vi "DefenderNormal.vi"(4 "Enemy Robots":T1, 5 "total":i32, 6 "balls":T4[](array[typedef]), 7 "cont old":dbl, 8 "ball old":dbl[](array[numeric]), 9 "Field Size in":T5, 10 "Numeric":i32, 11 "Our Robot in":T1) -> (1 "cont new":dbl, 2 "new ball":dbl[](array[numeric]), 3 "Robot out":T1)   [LabVIEW 2016]
uses:
  Core/AI Robot.ctl
  Functions Enum.ctl
  Core/Field Size.ctl
  Core/AI Ball.ctl
  <vilib>/Analysis/Matrix/Datatypes/RealMatrix.ctl
  <vilib>/Analysis/NI_AALBase.lvlib
  <vilib>/Analysis/baseanly.llb/Real A x B.vi
  <vilib>/Analysis/Matrix/NI_Matrix.lvlib
panel:
  in  "min dist to kick":dbl=195.0 format="%#_13g"
  in  "D max":dbl=400.0
  in  "D min":dbl=400.0
  in  "array":dbl[](array[numeric])
  out "fora?":bool
  in  "matrix":T3
  in  "y":dbl
  in  "raio robo":dbl=-90.0 format="%#_13g"
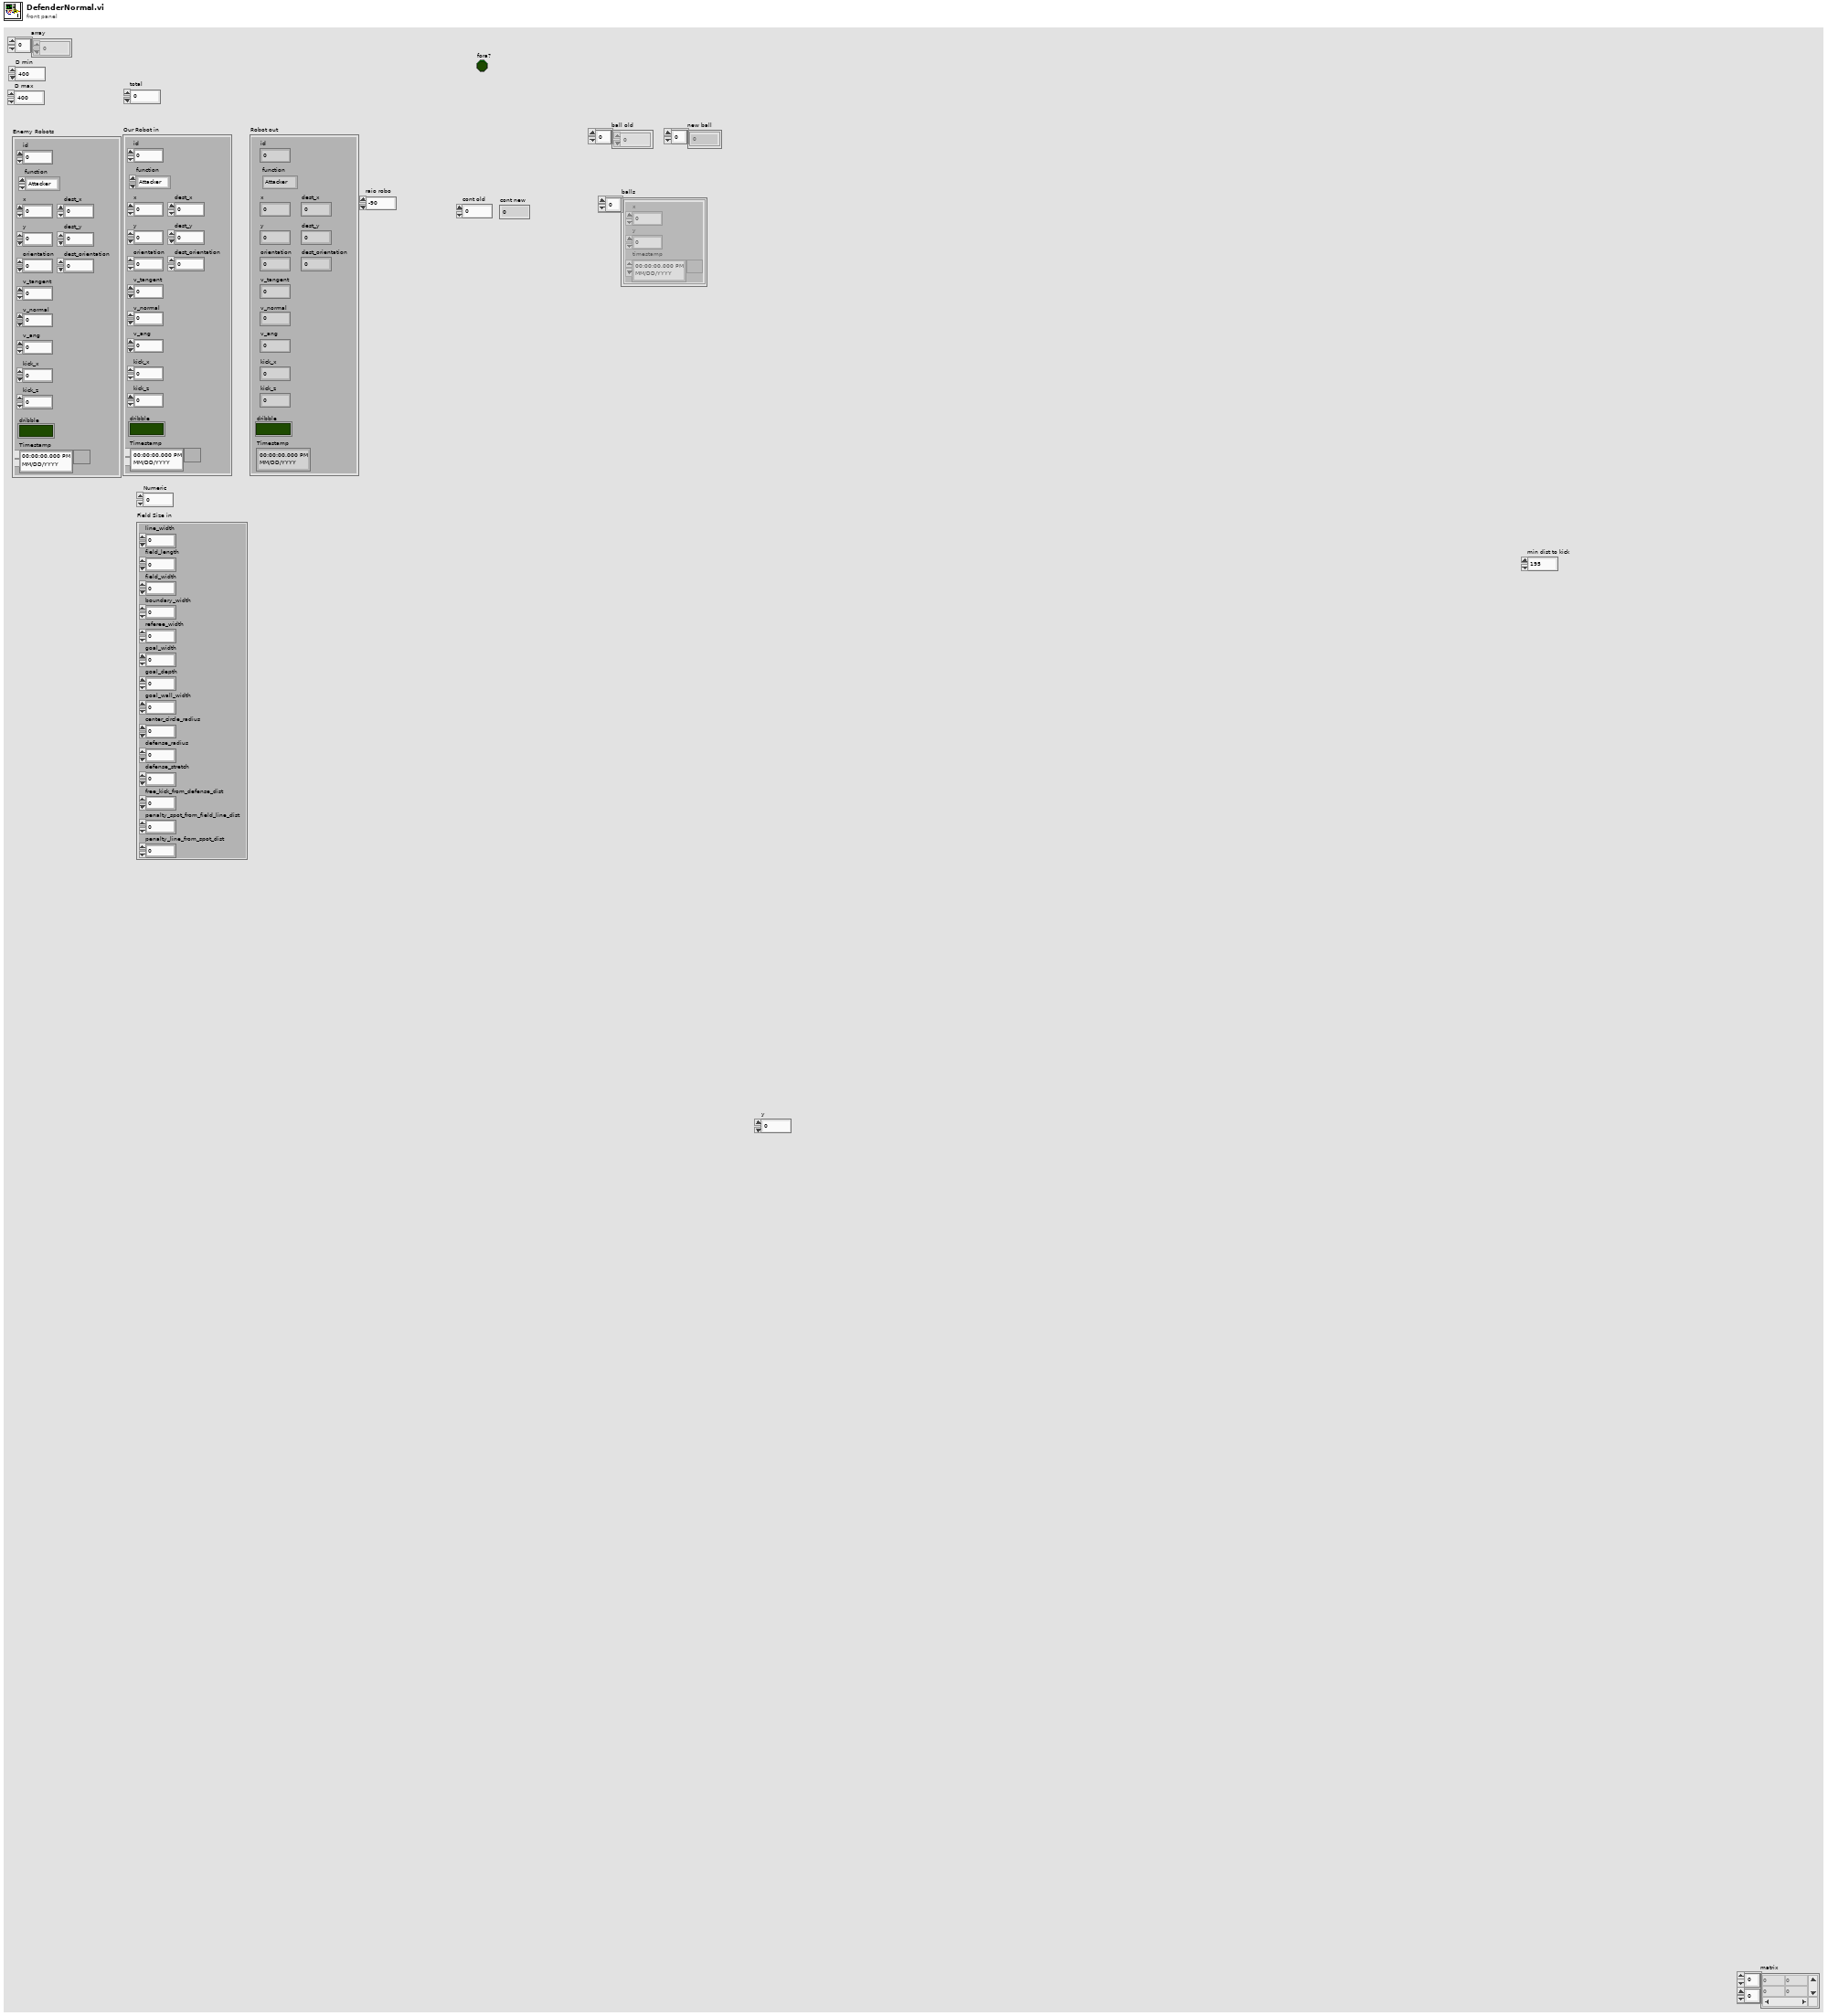
[diagram p1: front panel]
types:
  T1 = typedef "AI Robot.ctl" = cluster{"id":u32, "function":T2, "x":dbl, "y":dbl, "orientation":dbl, "v_tangent":dbl, "v_normal":dbl, "v_ang":dbl, "kick_x":dbl, "kick_z":dbl, "dribble":bool, "Timestamp":timestamp, "dest_x":dbl, "dest_y":dbl, "dest_orientation":dbl}
  T2 = typedef "Functions Enum.ctl" = enum16{"Attacker", "Goalie", "Defender", "Striker", "Goto 0", "Dummy", "ZigZag"}
  T3 = typedef "NI_Matrix.lvlib/RealMatrix.ctl" = dbl[][]
  T4 = typedef "AI Ball.ctl" = cluster{"x":dbl, "y":dbl, "timestamp":timestamp}
  T5 = typedef "Field Size.ctl" = cluster{"line_width":u32, "field_length":u32, "field_width":u32, "boundary_width":u32, "referee_width":u32, "goal_width":u32, "goal_depth":u32, "goal_wall_width":u32, "center_circle_radius":u32, "defense_radius":u32, "defense_stretch":u32, "free_kick_from_defense_dist":u32, "penalty_spot_from_field_line_dist":u32, "penalty_line_from_spot_dist":u32}
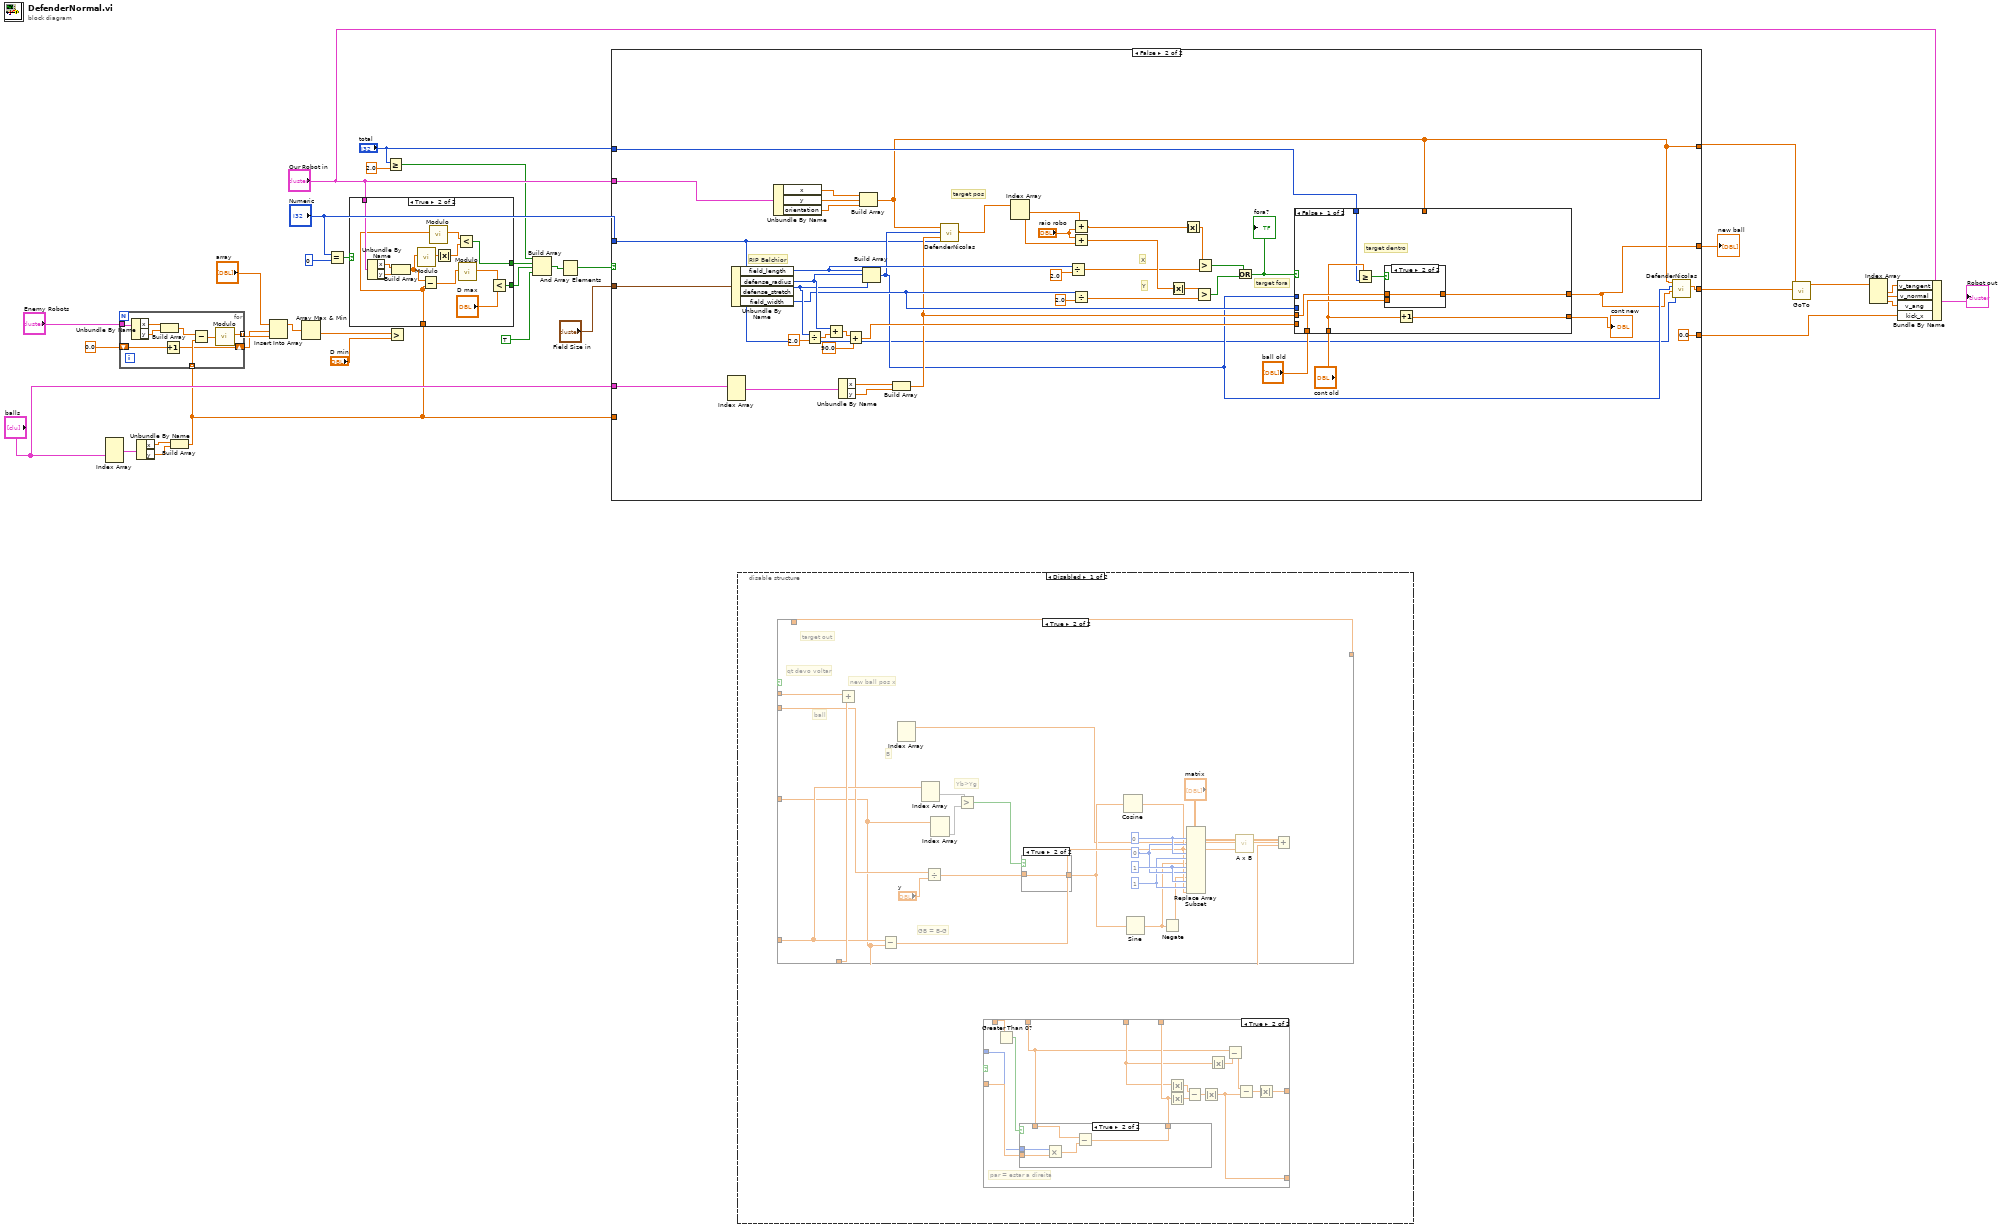
[diagram p0: block diagram]
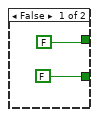
[diagram p2: hidden frame]
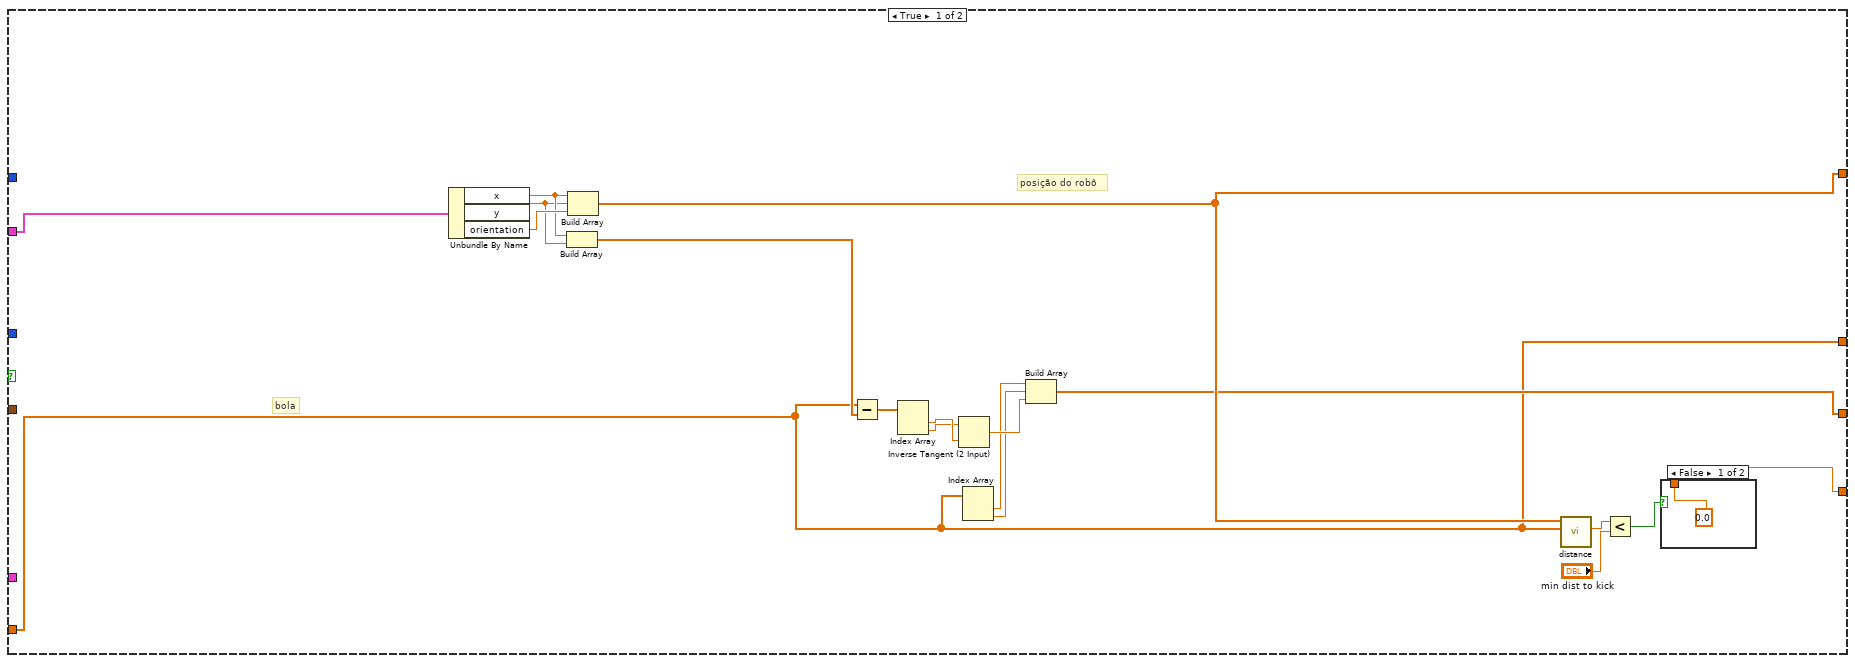
[diagram p3: hidden frame]
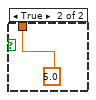
[diagram p4: hidden frame]
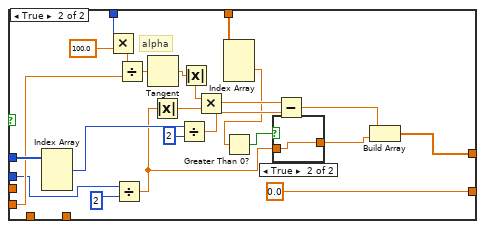
[diagram p6: hidden frame]
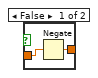
[diagram p7: hidden frame]
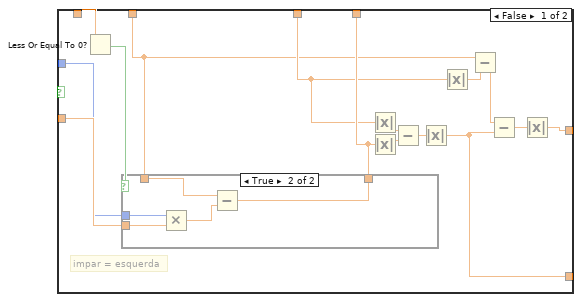
[diagram p8: hidden frame]
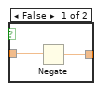
[diagram p12: hidden frame]
diagram:
  n1 = Index Array(array="balls") -> (element #1=w28:T4)  [unwired: 3 in, 2 out]
  n2 = Unbundle By Name(w28) -> ("x"=w5:dbl, "y"=w27:dbl)
  n3 = Build Array(w5, w27) -> (w6:dbl[])
  n4 = for {
    tunnel: "Enemy Robots" -> [w44]
    tunnel: w6 -> [w39] mode=indexing
    tunnel: [w38] -> w12 mode=indexing
    shift-right: [w36] -> w10
    shift-left: 0.0 -> [w37]
    n5 = Unbundle By Name(w44) -> ("x"=w43:dbl, "y"=w42:dbl)
    n6 = Build Array(w43, w42) -> (w41:dbl[])
    n7 = Increment(x=w37) -> (x+1=w36:dbl)
    n8 = Subtract(x=w41, y=w39) -> (x-y=w40:dbl[])
    n9 = call "Modulo.vi"("2D vector"=w40) -> ("Modulo"=w38:dbl)  [unwired: 10 in]
  }
  n10 = Insert Into Array(array="array", index=w10, new element=w12) -> (w9:dbl[])
  n11 = Array Max & Min(array=w9) -> (min value=w8:dbl)  [unwired: 3 out]
  n12 = Equal?(x="Numeric", y=0) -> (x = y?=w22:bool)
  n13 = case shown="True" w22 {
    tunnel: "Our Robot in" -> [_ w59]
    tunnel: [FALSE w55] -> w19
    tunnel: w6 -> [_ w49]
    tunnel: [FALSE w51] -> w3
    frame False {
    }
    frame True {
      n14 = Unbundle By Name(w59) -> ("x"=w53:dbl, "y"=w58:dbl)
      n15 = Build Array(w53, w58) -> (w47:dbl[])
      n16 = call "Modulo.vi"("2D vector"=w47) -> ("Modulo"=w48:dbl)  [unwired: 10 in]
      n17 = Subtract(x=w47, y=w49) -> (x-y=w54:dbl[])
      n18 = call "Modulo.vi"("2D vector"=w49) -> ("Modulo"=w50:dbl)  [unwired: 10 in]
      n19 = Absolute Value(x=w48) -> (abs(x)=w52:dbl)
      n20 = Less?(x=w50, y=w52) -> (x < y?=w51:bool)
      n21 = call "Modulo.vi"("2D vector"=w54) -> ("Modulo"=w57:dbl)  [unwired: 10 in]
      n22 = Less?(x=w57, y="D max") -> (x < y?=w55:bool)
    }
  }
  n23 = Greater Or Equal?(x="total", y=2.0) -> (x >= y?=w4:bool)
  n24 = Greater?(x=w8, y="D min") -> ()  [unwired: 1 out]
  n25 = Build Array(w4, w3, w19, TRUE ("element")) -> (w18:bool[])
  n26 = And Array Elements(Boolean array=w18) -> (logical AND=w17:bool)
  n27 = case shown="False" w17 {
    tunnel: "Our Robot in" -> [w61 w112]
    tunnel: "Field Size in" -> [_ w110]
    tunnel: "balls" -> [_ w102]
    tunnel: [w64 w80] -> w30
    tunnel: "Numeric" -> [_ w81]
    tunnel: [w73 w84] -> w29
    tunnel: "total" -> [_ w89]
    tunnel: [w74 0.0] -> w16
    tunnel: w6 -> [w60 _]
    tunnel: [w60 w82] -> w2
    frame True {
      # "posição do robô"
      # "bola"
      n28 = Unbundle By Name(w61) -> ("x"=w71:dbl, "y"=w70:dbl, "orientation"=w72:dbl)
      n29 = Build Array(w71, w70) -> (w69:dbl[])
      n30 = Build Array(w71, w70, w72) -> (w73:dbl[])
      n31 = Subtract(x=w60, y=w69) -> (x-y=w68:dbl[])
      n32 = Index Array(array=w68) -> (element #1=w66:dbl, element #2=w65:dbl)  [unwired: 2 in]
      n33 = Inverse Tangent (2 Input)(1:w66, 2:w65) -> (0:w67:dbl)
      n34 = Index Array(array=w60) -> (element #1=w63:dbl, element #2=w62:dbl)  [unwired: 2 in]
      n35 = Build Array(w63, w62, w67) -> (w64:dbl[])
      n36 = call "distance.vi"("target pos"=w60, "obj pos"=w73) -> ("sqrt(x)"=w77:dbl)  [unwired: 9 in]
      n37 = Less?(x=w77, y="min dist to kick") -> (x < y?=w76:bool)
      n38 = case shown="False" w76 {
        tunnel: [0.0 5.0] -> w74
        frame False {
        }
        frame True {
        }
      }
    }
    frame False {
      # "RIP Belchior"
      # "target fora"
      # "Y"
      # "X"
      # "target pos"
      n39 = Index Array(array=w102) -> (element #1=w123:T4)  [unwired: 3 in, 2 out]
      n40 = Unbundle By Name(w110) -> ("field_length"=w107:u32, "defense_radius"=w97:u32, "defense_stretch"=w94:u32, "field_width"=w90:u32)
      n41 = Unbundle By Name(w112) -> ("x"=w108:dbl, "y"=w104:dbl, "orientation"=w103:dbl)
      n42 = Divide(x=w94, y=2.0) -> (x/y=w95:dbl)
      n43 = Add(x=w97, y=w95) -> (x+y=w92:dbl)
      n44 = Unbundle By Name(w123) -> ("x"=w113:dbl, "y"=w109:dbl)
      n45 = Add(x=w92, y=90.0) -> (x+y=w93:dbl)
      n46 = Build Array(w108, w104, w103) -> (w84:dbl[])
      n47 = Build Array(w107, w97, w94) -> (w83:u32[])
      n48 = Build Array(w113, w109) -> (w86:dbl[])
      n49 = call "DefenderNicolas.vi"("R"=w84, "Field"=w83, "Ball"=w86, "Numeric"=w81) -> ("target"=w85:dbl[])  [unwired: 6 in]
      n50 = Index Array(array=w85) -> (element #1=w106:dbl, element #2=w105:dbl)  [unwired: 2 in]
      n51 = Divide(x=w107, y=2.0) -> (x/y=w101:dbl)
      n52 = Add(x=w106, y="raio robo") -> (x+y=w111:dbl)
      n53 = Add(x="raio robo", y=w105) -> (x+y=w114:dbl)
      n54 = Divide(x=w90, y=2.0) -> (x/y=w116:dbl)
      n55 = Absolute Value(x=w114) -> (abs(x)=w119:dbl)
      n56 = Absolute Value(x=w111) -> (abs(x)=w120:dbl)
      n57 = Greater?(x=w119, y=w116) -> (0:w117:bool)
      n58 = Greater?(x=w120, y=w101) -> (0:w118:bool)
      n59 = Or(x=w118, y=w117) -> (x .or. y?=w100:bool)
      "fora?" <- w100
      n60 = case shown="False" w100 {
        tunnel: w86 -> [w128 _]
        tunnel: [w129 w152] -> w82
        tunnel: "ball old" -> [w127 _]
        tunnel: "cont old" -> [w125 _]
        tunnel: [w130 0.0] -> w98
        tunnel: w83 -> [_ w154]
        tunnel: w93 -> [_ w148]
        tunnel: w89 -> [w124 w151]
        tunnel: w90 -> [_ w141]
        tunnel: w84 -> [_ w137]
        frame False {
          # "target dentro"
          n61 = Greater Or Equal?(x=w125, y=w124) -> (x >= y?=w126:bool)
          n62 = case shown="True" w126 {
            tunnel: [w131 w132] -> w129
            tunnel: w128 -> [_ w132]
            tunnel: w127 -> [w131 _]
            frame False {
            }
            frame True {
            }
          }
          n63 = Increment(x=w125) -> (x+1=w130:dbl)
        }
        frame True {
          # "alpha"
          n64 = Index Array(array=w154) -> (element #1=w139:u32)  [unwired: 3 in, 2 out]
          n65 = Multiply(x=w151, y=100.0) -> (x*y=w149:dbl)
          n66 = Divide(x=w141, y=u32 2) -> (x/y=w134:dbl)
          n67 = Divide(x=w149, y=w148) -> (x/y=w146:dbl)
          n68 = Tangent(1:w146) -> (0:w145:dbl)
          n69 = Absolute Value(x=w134) -> (abs(x)=w144:dbl)
          n70 = Divide(x=w139, y=u32 2) -> (x/y=w140:dbl)
          n71 = Absolute Value(x=w145) -> (abs(x)=w147:dbl)
          n72 = Multiply(x=w147, y=w144) -> (x*y=w143:dbl)
          n73 = Index Array(array=w137) -> (element #2=w136:dbl)  [unwired: 3 in, 2 out]
          n74 = Greater Than 0?(x=w136) -> (x > 0?=w135:bool)
          n75 = case shown="True" w135 {
            tunnel: w134 -> [w157 w158]
            tunnel: [w156 w158] -> w133
            frame False {
              n76 = Negate(x=w157) -> (-x=w156:dbl)
            }
            frame True {
            }
          }
          n77 = Subtract(x=w143, y=w140) -> (x-y=w142:dbl)
          n78 = Build Array(w142, w133) -> (w152:dbl[])
        }
      }
      "cont new" <- w98
      n79 = call "DefenderNicolas.vi"("R"=w84, "Field"=w83, "Ball"=w82, "Numeric"=w81) -> ("target"=w80:dbl[])  [unwired: 6 in]
    }
  }
  "new ball" <- w2
  n80 = disable-structure shown="Disabled" {
    frame Disabled {
      n81 = case shown="True" {
        selector: _ -> [_ _]
        tunnel: _ -> [_ w225]
        tunnel: _ -> [_ w224]
        tunnel: _ -> [_ w206]
        tunnel: _ -> [_ w207]
        tunnel: _ -> [_ w204]
        tunnel: [w201 w202] -> _
        tunnel: _ -> [w201 w202]
        frame False {
        }
        frame True {
          w220 = 1
          w221 = 0
          w222 = 1
          w223 = 0
          # "B"
          # "Yb>Yg"
          # "GB = B-G"
          # "new ball pos x"
          # "qt devo voltar"
          # "ball"
          # "target out"
          n82 = Add(x=w224, y=w225) -> ()  [unwired: 1 out]
          n83 = Subtract(x=w207, y=w204) -> (x-y=w215:dbl)
          n84 = Index Array(array=w207) -> (element #2=w214)  [unwired: 2 in, 1 out]
          n85 = Divide(x=w206, y="y") -> (x/y=w211:dbl)
          n86 = Index Array(array=w204) -> (element #2=w213)  [unwired: 2 in, 1 out]
          n87 = Greater?(x=w214, y=w213) -> (0:w212:bool)
          n88 = case shown="True" w212 {
            tunnel: [w226 w228] -> w210
            tunnel: w211 -> [w227 w228]
            frame False {
              n89 = Negate(x=w227) -> (-x=w226:dbl)
            }
            frame True {
            }
          }
          n90 = Cosine(x=w210) -> (cos(x)=w219:dbl)
          n91 = Sine(x=w210) -> (sin(x)=w217:dbl)
          n92 = Negate(x=w217) -> (-x=w218:dbl)
          n93 = Replace Array Subset(array="matrix", new element #1=w219, index (row) #1=w223, index (col) #1=w221, new element #2=w217, index (row) #2=w223, index (col) #2=w220, new element #3=w218, index (row) #3=w222, index (col) #3=w221, new element #4=w219, index (row) #4=w222, index (col) #4=w220) -> (w208:T3)
          n94 = call-poly <vilib>:"A x B.vi"("B"=w215, "A"=w208) -> ("A x B"=w209:T3)  [unwired: 1 out]
          n95 = Add ("Add.vi")(x=w209, y=w204) -> (x+y=w203:dbl)
          n96 = Index Array(array=w203) -> ()  [unwired: 2 in, 2 out]
        }
      }
      n97 = case shown="True" {
        selector: _ -> [_ _]
        tunnel: _ -> [w173 w194]
        tunnel: _ -> [w160 w181]
        tunnel: [w166 w187] -> _
        tunnel: _ -> [w171 w192]
        tunnel: _ -> [w170 w191]
        tunnel: _ -> [w162 w186]
        tunnel: [w161 w182] -> _
        tunnel: [w159 w180] -> _
        frame False {
          # "impar = esquerda"
          n98 = Less Or Equal To 0?(x=w173) -> (x <= 0?=w172:bool)
          n99 = case shown="True" w172 {
            tunnel: [w174 w175] -> w166
            tunnel: w160 -> [w174 w176]
            tunnel: w171 -> [_ w178]
            tunnel: w170 -> [_ w177]
            frame False {
            }
            frame True {
              n100 = Multiply(x=w177, y=w178) -> (x*y=w179:dbl)
              n101 = Subtract(x=w176, y=w179) -> (x-y=w175:dbl)
            }
          }
          n102 = Absolute Value(x=w162) -> (abs(x)=w168:dbl)
          n103 = Absolute Value(x=w166) -> (abs(x)=w167:dbl)
          n104 = Subtract(x=w168, y=w167) -> (x-y=w169:dbl)
          n105 = Absolute Value(x=w169) -> (abs(x)=w159:dbl)
          n106 = Absolute Value(x=w162) -> (abs(x)=w163:dbl)
          n107 = Subtract(x=w160, y=w163) -> (x-y=w164:dbl)
          n108 = Subtract(x=w164, y=w159) -> (x-y=w165:dbl)
          n109 = Absolute Value(x=w165) -> (abs(x)=w161:dbl)
        }
        frame True {
          # "par = estar a direita"
          n110 = Greater Than 0?(x=w194) -> (x > 0?=w193:bool)
          n111 = case shown="True" w193 {
            tunnel: w181 -> [w195 w199]
            tunnel: [w195 w200] -> w187
            tunnel: w192 -> [_ w197]
            tunnel: w191 -> [_ w196]
            frame False {
            }
            frame True {
              n112 = Multiply(x=w196, y=w197) -> (x*y=w198:dbl)
              n113 = Subtract(x=w199, y=w198) -> (x-y=w200:dbl)
            }
          }
          n114 = Absolute Value(x=w186) -> (abs(x)=w189:dbl)
          n115 = Absolute Value(x=w187) -> (abs(x)=w188:dbl)
          n116 = Subtract(x=w189, y=w188) -> (x-y=w190:dbl)
          n117 = Absolute Value(x=w190) -> (abs(x)=w180:dbl)
          n118 = Absolute Value(x=w186) -> (abs(x)=w185:dbl)
          n119 = Subtract(x=w181, y=w185) -> (x-y=w184:dbl)
          n120 = Subtract(x=w184, y=w180) -> (x-y=w183:dbl)
          n121 = Absolute Value(x=w183) -> (abs(x)=w182:dbl)
        }
      }
    }
    frame Enabled {
    }
  }
  n122 = call "GoTo.vi"("Target"=w30, "Position"=w29) -> ("Output\nVelocity"=w33:dbl[])  [unwired: 8 in, 1 out]
  n123 = Index Array(array=w33) -> (element #1=w1:dbl, element #2=w34:dbl, element #3=w35:dbl)  [unwired: 3 in]
  n124 = Bundle By Name(cluster="Our Robot in", "v_tangent"=w1, "v_normal"=w34, "v_ang"=w35, "kick_x"=w16) -> (→"Robot out":T1)
